vi "Labview and Arduino UNO Based Fire Detection Motinoring.vi"() -> ()   [LabVIEW 2018]
uses:
  <vilib>/MakerHub/LINX/Public/Peripherals/Digital/Digital Read 1 Chan.vi
  <vilib>/MakerHub/LINX/Public/Peripherals/Analog/Analog Read 1 Chan.vi
  <vilib>/MakerHub/LINX/Public/Peripherals/Digital/Digital Read N Chans.vi
  <vilib>/MakerHub/LINX/Public/Peripherals/Analog/Analog Read N Chans.vi
  <vilib>/MakerHub/LINX/Private/Local IO/LinxDigitalRead.vi
  <vilib>/MakerHub/LINX/Public/Utilities/Check Channel.vi
  <vilib>/MakerHub/LINX/Private/Local IO/LinxAnalogRead.vi
  <vilib>/MakerHub/LINX/Public/Utilities/Open Serial.vi
  <vilib>/MakerHub/LINX/Private/Utilties/Generate Error.vi
  <vilib>/MakerHub/LINX/LMH-LINX.lvlib
panel:
  in  "Voltage Ajustment":dbl(knob) scale=0.0..5.0
  out "AI Ref":dbl
  out "Voltage":dbl
  out "Device Name":string
  in  "?":bool
  out "Waveform Chart":i16(graph)
  in  "Serial Port":refnum<visa-resource-name>="N/A"
  # "LABVIEW AND ARDUINO UNO BASED FIRE DETECTION MOTINORING"
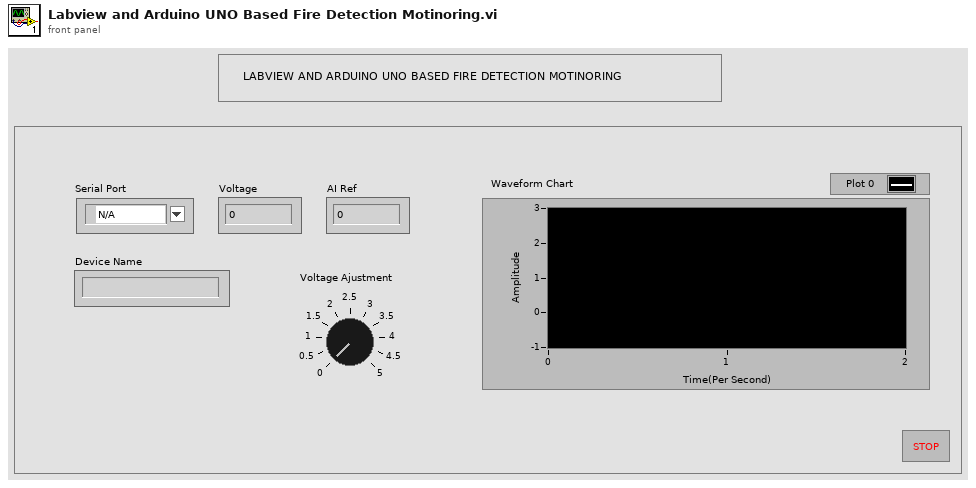
[diagram p1: front panel]
types:
  T1 = typedef "LMH-LINX.lvlib/LINX Ref.ctl" = cluster{"IO":T2, "Interface":T3, "LINX Device Config":T4}
  T2 = typedef "LMH-LINX.lvlib/Platform.ctl" = enum16{"Remote", "Local"}
  T3 = typedef "LMH-LINX.lvlib/Interface.ctl" = enum16{"Serial", "TCP"}
  T4 = typedef "LMH-LINX.lvlib/Device.lvlib/LINX Device Config.ctl" = cluster{"Interface":T3, "COM Port":refnum<visa-resource-name>, "TCP Configuration":T5, "Device Family":u8, "Device ID":u8, "Device Name":string, "TCP Ref":refnum<k5>, "Channels":T6}
  T5 = typedef "LMH-LINX.lvlib/Device.lvlib/TCP Config.ctl" = cluster{"IP Address":string, "Port":u16}
  T6 = typedef "LMH-LINX.lvlib/Channels.ctl" = cluster{"DI":u8[], "DO":u8[], "AI":u8[], "AO":u8[], "PWM":u8[], "QE":u8[], "UART":u8[], "I2C 2":u8[], "SPI":u8[], "CAN":u8[], "Servo":u8[], "AI Ref (V)":dbl, "AI Resolution (Bits)":u8, "AO Ref (V)":dbl, "AO Resolution (Bits)":u8}
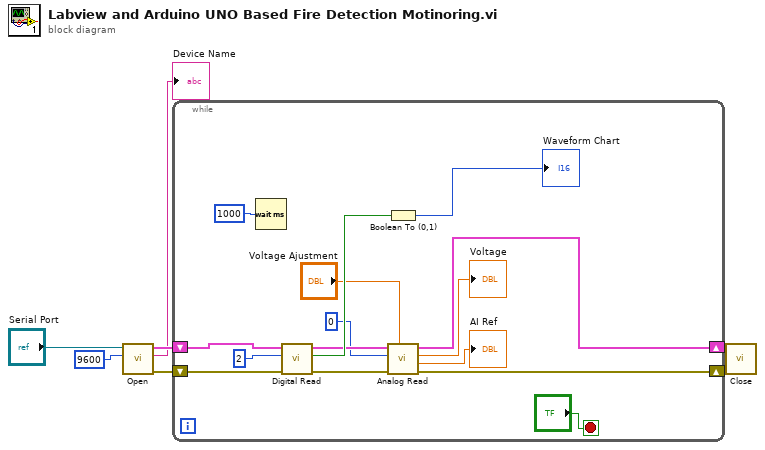
[diagram p0: block diagram]
diagram:
  n1 = call-poly <vilib>:"Open.vi"("Baud Rate Override"=u32 9600, "Serial Port"="Serial Port") -> ("Error Out"=w6:errorcluster, "Device Name"=→"Device Name":string, "LINX Resource"=w7:T1)  [unwired: 7 in]
  n2 = while {
    shift-right: [w8] -> w5
    shift-left: w7 -> [w22]
    shift-right: [w13] -> w4
    shift-left: w6 -> [w21]
    stop <- "?" stop-if-true
    n3 = Wait (ms)(milliseconds to wait=u32 1000) -> ()  [unwired: 1 out]
    n4 = call-poly <vilib>:"Digital Read.vi"("Error In"=w21, "DI Channel"=u8 2, "LINX Resource"=w22) -> ("Error Out"=w14:errorcluster, "DI Value"=w16:bool, "LINX Resource"=w15:T1)  [unwired: 6 in]
    n5 = Boolean To (0,1)(Boolean=w16) -> (0, 1=→"Waveform Chart":i16)
    n6 = call-poly <vilib>:"Analog Read.vi"("Analog Ref Override (V)"="Voltage Ajustment", "Error In"=w14, "Analog Channel"=u8 0, "LINX Resource"=w15) -> ("Error Out"=w13:errorcluster, "AI Ref"=→"AI Ref":dbl, "Voltage"=→"Voltage":dbl, "LINX Resource"=w8:T1)  [unwired: 4 in]
  }
  n7 = call <vilib>:"Close.vi"("Error In"=w4, "LINX Resource"=w5) -> ()  [unwired: 9 in, 1 out]
